vi "NicmosTemperatureControl.vi"(7 "error in (no error)":errorcluster caption="entrée d'erreur") -> (0 "T2":dbl format="%.2f", 1 "T1":dbl format="%.2f", 4 "error out":errorcluster caption="sortie d'erreur")   [LabVIEW 2009]
uses:
  <vilib>/Analysis/NI_AALBase.lvlib
panel:
  out "Numérique":i32
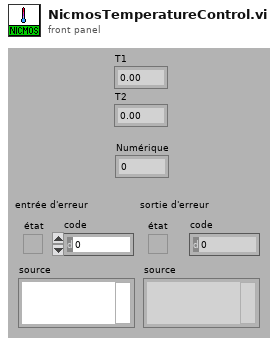
[diagram p1: front panel]
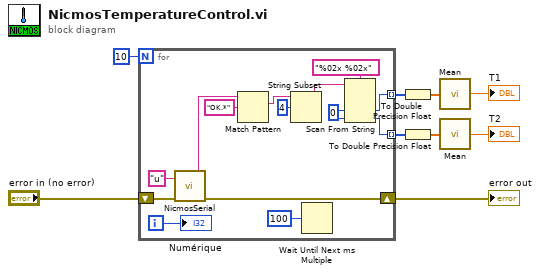
[diagram p0: block diagram]
diagram:
  n1 = for {
    N: 10 -> [_]
    tunnel: [w18] -> w9 mode=indexing
    tunnel: [w17] -> w8 mode=indexing
    shift-right: [w12] -> w7
    shift-left: "error in (no error)" -> [w13]
    i -> [w11]
    w16 = 0 ("Valeur par défaut1")
    n2 = call "NicmosSerial.vi"("error in"=w13, "Command"="u") -> ("error out"=w12:errorcluster, "Answer"=w22:string)  [unwired: 3 in]
    n3 = Match Pattern(string=w22, regular expression="OK.*" ("expression")) -> (match substring=w14:string)  [unwired: 1 in, 3 out]
    n4 = String Subset(string=w14, offset (0)=4) -> (substring=w15:string)  [unwired: 1 in]
    n5 = Wait Until Next ms Multiple(millisecond multiple=u32 100 ("n millisecondes")) -> ()  [unwired: 1 out]
    n6 = Scan From String(format string="%02x %02x" ("Chaîne de format"), input string=w15, default 1=w16, default 2=w16) -> (output 1=w18:i32, output 2=w17:i32)  [unwired: 2 in, 3 out]
    "Numérique" <- w11
  }
  "error out" <- w7
  n7 = To Double Precision Float(number=w9) -> (double precision float=w6:dbl[])
  n8 = To Double Precision Float(number=w8) -> (double precision float=w5:dbl[])
  n9 = call <vilib>:"Mean.vi"("X"=w6) -> ("mean"=→"T1":dbl)  [unwired: 1 out]
  n10 = call <vilib>:"Mean.vi"("X"=w5) -> ("mean"=→"T2":dbl)  [unwired: 1 out]
